vi "sip.vi"() -> ()   [LabVIEW 2020]
uses:
  <vilib>/Instr/_visa.llb/VISA Configure Serial Port (Instr).vi
panel:
  in  "stop":bool
  out "read buffer":string
  in  "VISA resource name":refnum<visa-resource-name>
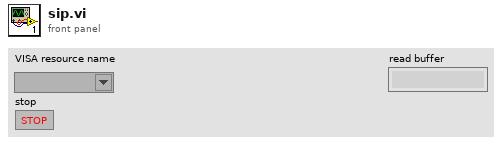
[diagram p1: front panel]
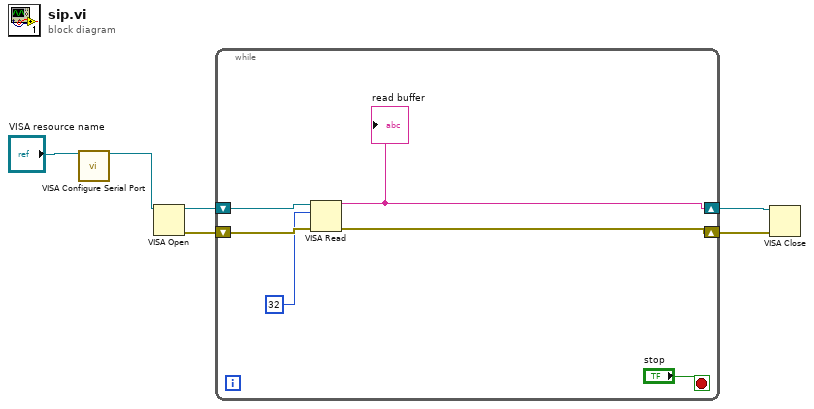
[diagram p0: block diagram]
diagram:
  n1 = call-poly "VISA Configure Serial Port"("VISA resource name"="VISA resource name") -> ("VISA resource name out"=w5:refnum<visa-resource-name>)  [unwired: 13 in, 1 out]
  n2 = VISA Open(VISA resource name=w5) -> (VISA resource name=w4:refnum<visa-resource-name>, error out=w3:errorcluster)  [unwired: 4 in]
  n3 = while {
    shift-right: [w10] -> w2
    shift-left: w4 -> [w12]
    shift-right: [w9] -> w1
    shift-left: w3 -> [w11]
    stop <- "stop" stop-if-true
    n4 = VISA Read(VISA resource name=w12, byte count=u32 32, error in (no error)=w11) -> (read buffer=w10:string, error out=w9:errorcluster)  [unwired: 2 out]
    "read buffer" <- w10
  }
  n5 = VISA Close(VISA resource name=w2, error in (no error)=w1) -> ()  [unwired: 1 out]
